vi "Open Connection.vi"(8 "error in (no error)":errorcluster, 10 "Connection string":string, 11 "IDatabase in":refnum<class "IDatabase.lvclass">) -> (0 "error out":errorcluster, 3 "IDatabase out":refnum<class "IDatabase.lvclass">)   [LabVIEW 2020, in "IDatabase.lvlib" / "IDatabase.lvclass"]
uses:
  IDatabase.lvclass
  <vilib>/Utility/error.llb/Error Cluster From Error Code.vi
  <vilib>/ErrorRing/Error Ring.xnode
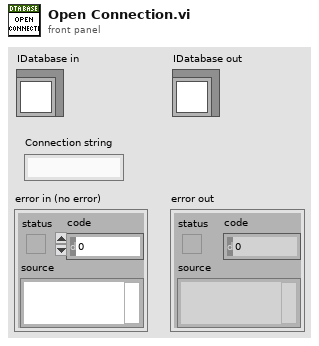
[diagram p1: front panel]
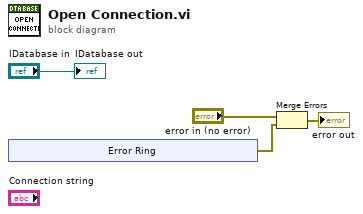
[diagram p0: block diagram]
diagram:
  n1 = xnode "Error Ring"() -> ("error out"=w2:errorcluster)
  n2 = Merge Errors("error in (no error)", w2) -> (→"error out":errorcluster)
  "IDatabase out" <- "IDatabase in"
